vi "NEW TESTS 4 channel fixed pixel clock resonance scanner acquisition (Host).vi"() -> ()   [LabVIEW 2012]
uses:
  <vilib>/rvi/interface/nirviOpenFPGA/nirviOpenFPGA.xnode
  <vilib>/rvi/interface/nirviMethod/nirviMethod.xnode
  <vilib>/rvi/interface/nirviReadWriteControl/nirviReadWriteControl.xnode
  <vilib>/rvi/errors/niLvFpgaMergeErrorWithErrorCode.vi
  <vilib>/rvi/interface/nirviCloseFPGA/nirviCloseFPGA.xnode
  <vilib>/DAQmx/create/channels.llb/DAQmx Create Channel (AO-Voltage-Basic).vi
  <vilib>/DAQmx/configure/timing.llb/DAQmx Timing (Sample Clock).vi
  <vilib>/DAQmx/write.llb/DAQmx Write (Analog 1D DBL 1Chan NSamp).vi
  <vilib>/DAQmx/configure/trigger.llb/DAQmx Start Trigger (Digital Edge).vi
  D/Dropbox/Scientifica SoftScan project/fpga testing/4 ch resonance scanner acquisition (FPGA) fixed pix clock.vi
  Scientifica SoftScan project/fpga testing/FPGA Bitfiles/4chresonancescan_PXIe-7962R_newLindsaymod4ch_VaUfink3TSc.lvbitx
  <vilib>/userdefined/High Color/nirio_resource_hc.ctl
panel:
  in  "Numeric":i32=200
  out "Waveform Graph 2":i32[](graph)
  out "Array 4":i32[](array[numeric])
  out "sum 2":i16
  out "Array 3":u32[](array[numeric])
  out "max index(es)":i32
  out "Waveform Graph":u32[](graph)
  out "min value":u32
  out "max value":u32
  out "avg value":dbl
  out "sum":u32
  out "Array 2":u32[](array[numeric])
  out "Array":u32[](array[numeric])
  out "Waveform Chart":u32[](graph)
  out "Timed Out":bool
  out "Numeric 2":i32
  in  "data":dbl=1.0
  in  "y-voltage":dbl=4.0
  out "error out":errorcluster
  in  "stop":bool
  in  "Requested Depth":u32=100000000
  in  "lines (2pi) per frame":i32=100
  out "Actual Depth 3":u32
  out "Actual Depth":u32
  in  "Start Delay (Ticks)":i16
  in  "RIO Device":T1="RIO0"
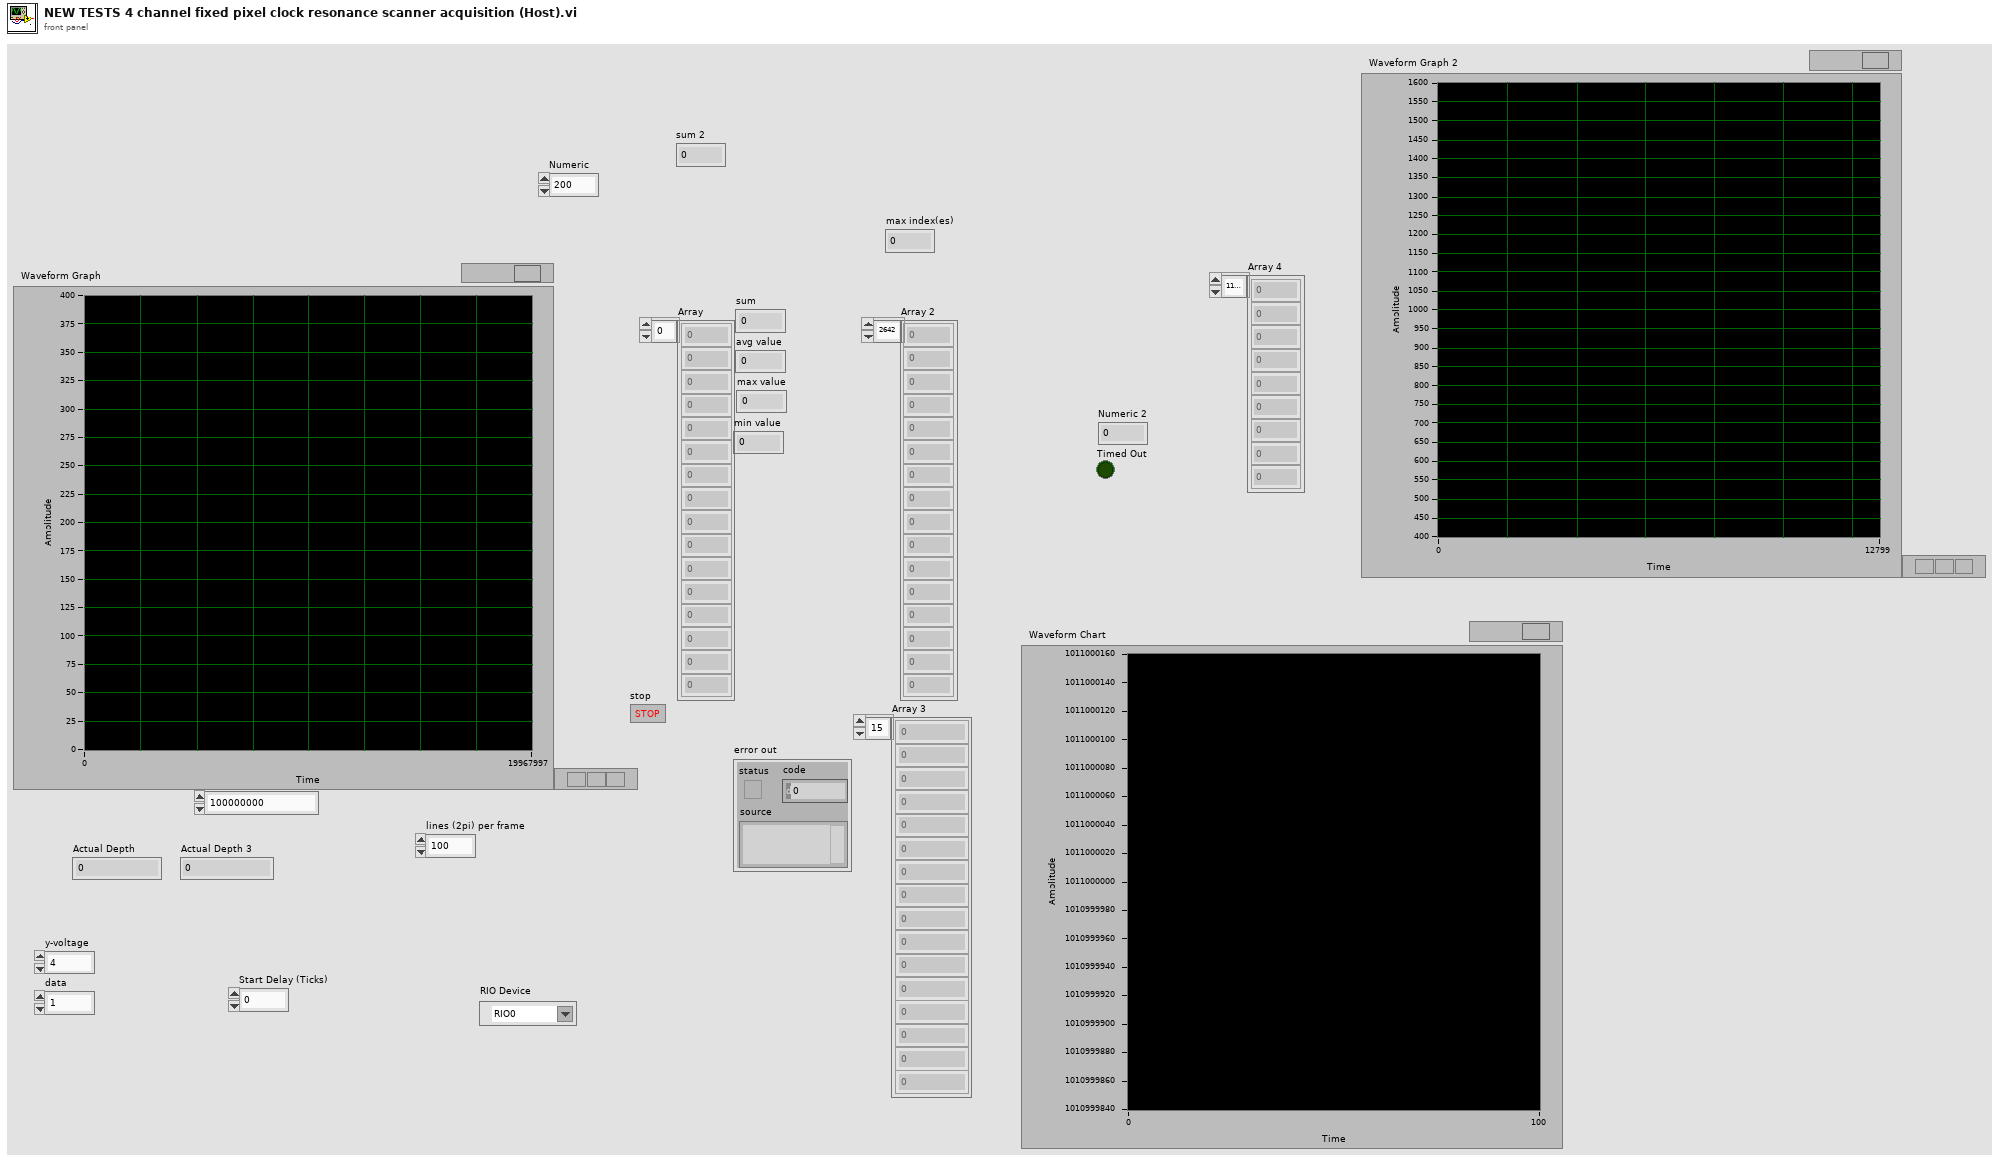
[diagram p1: front panel]
types:
  T1 = typedef "nirio_resource_hc.ctl" = tag
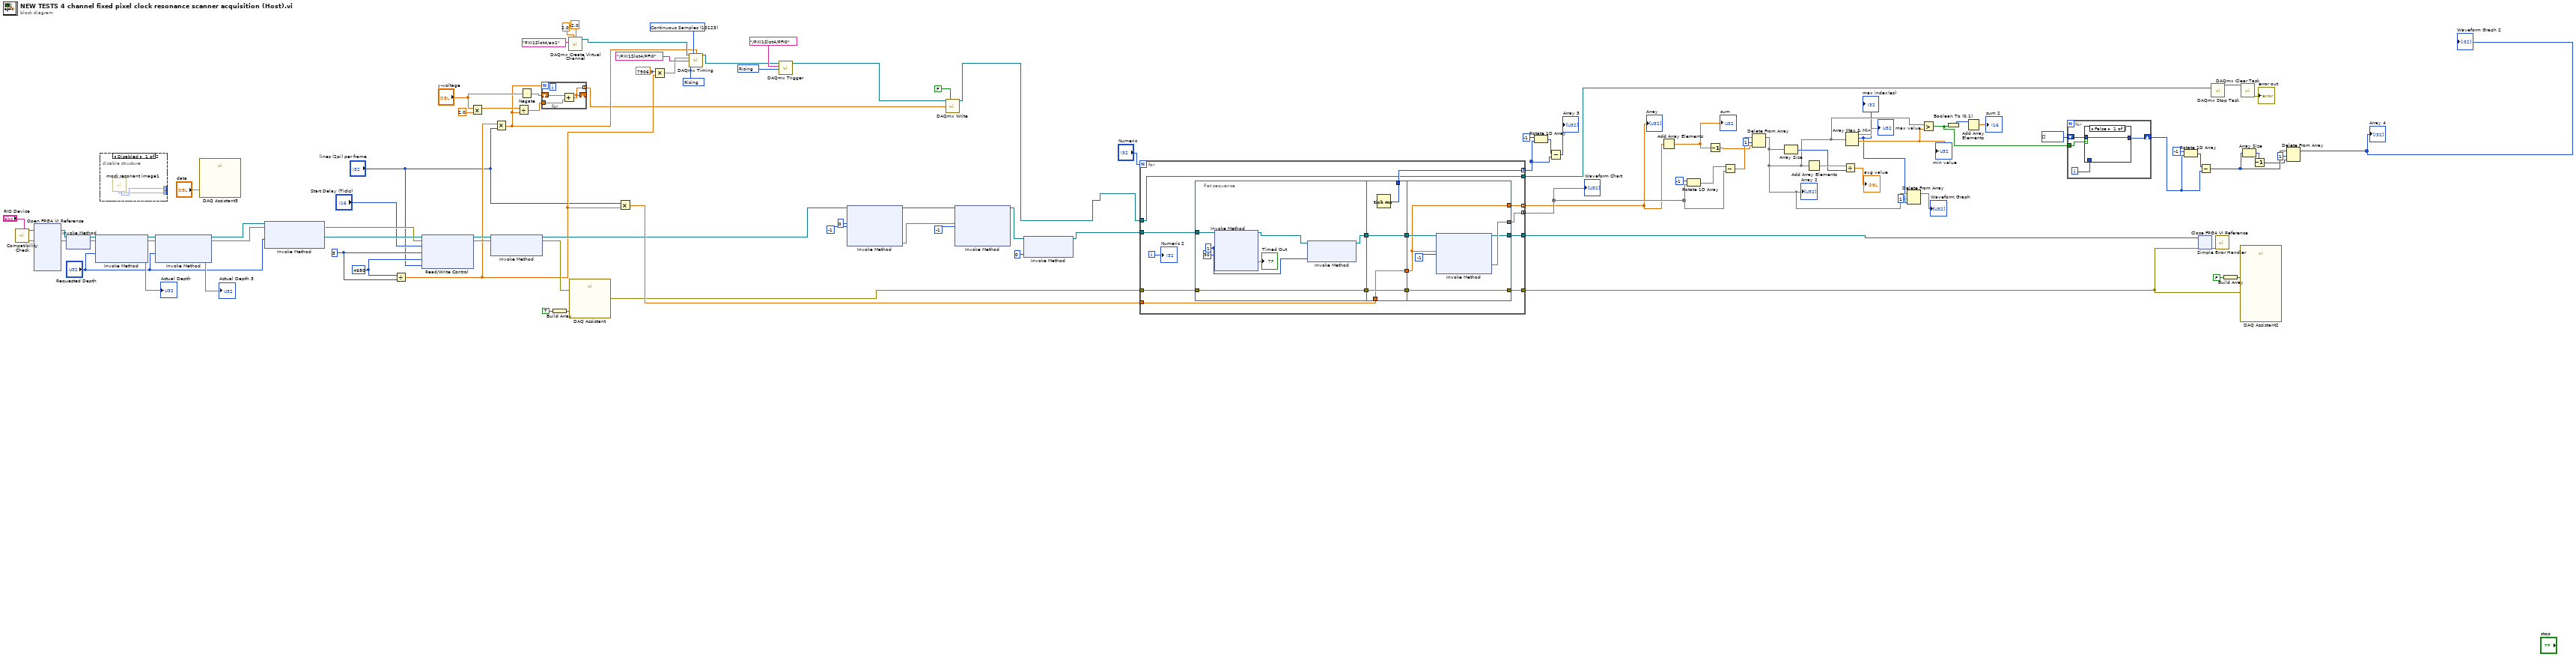
[diagram p0: block diagram]
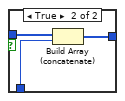
[diagram p2: hidden frame]
diagram:
  w10 = 10280 items=["Rising"=10280, "Falling"=10171] ("active edge")
  w75 = 10123 items=["Finite Samples"=10178, "Continuous Samples"=10123, "Hardware Timed Single Point"=12522] ("sample mode")
  w85 = 3 ("dwell time in ticks")
  w8 = i16 4680 ("samples per period")
  w89 = 10280 items=["Rising"=10280, "Falling"=10171] ("edge")
  n1 = call "Compatibility Check.vi"() -> ("error out"=w101:errorcluster)  [unwired: 2 in, 9 out]
  n2 = xnode "Open FPGA VI Reference"("error in"=w101, "resource name"="RIO Device") -> ("FPGA VI Reference Out"=w98:refnum<k20>, "error out"=w99:errorcluster)
  n3 = xnode "Invoke Method"("FPGA VI Reference In"=w98, "error in"=w99) -> ("FPGA VI Reference Out"=w97:refnum<k20>, "error out"=w88:errorcluster)
  n4 = xnode "Invoke Method"("FPGA VI Reference In"=w97, "error in"=w88, "Requested Depth"="Requested Depth") -> ("FPGA VI Reference Out"=w93:refnum<k20>, "error out"=w87:errorcluster, "Actual Depth"=→"Actual Depth")
  n5 = disable-structure shown="Disabled" {
    disable-tunnel: [w103 _] -> _
    disable-tunnel: [w102 _] -> _
    frame Disabled {
      n6 = call "mock resonant image1.vi"() -> ("samples per period (fix pix clock)"=w103:i32, "fixed dwell time"=w102:i32)  [unwired: 7 in, 3 out]
    }
    frame Enabled {
    }
  }
  n7 = xnode "Invoke Method"("FPGA VI Reference In"=w93, "error in"=w87, "Requested Depth"="Requested Depth") -> ("FPGA VI Reference Out"=w72:refnum<k20>, "error out"=w71:errorcluster, "Actual Depth"=→"Actual Depth 3")
  n8 = call "DAQ Assistant3"("data"="data") -> ()  [unwired: 17 in, 2 out]
  n9 = xnode "Invoke Method"("FPGA VI Reference In"=w72, "error in"=w71, "Requested Depth"="Requested Depth") -> ("FPGA VI Reference Out"=w70:refnum<k20>, "error out"=w69:errorcluster)  [unwired: 1 out]
  n10 = Divide(x=w8, y=w85) -> (x/y=w5:dbl)
  n11 = xnode "Read/Write Control"("FPGA VI Reference In"=w70, "error in"=w69, "Start Delay (Ticks)"="Start Delay (Ticks)", "dwell time in ticks"=w85, "samples per period"=w8, "lines at once"="lines (2pi) per frame") -> ("FPGA VI Reference Out"=w96:refnum<k20>, "error out"=w86:errorcluster)
  n12 = Multiply(x="y-voltage", y=2.0) -> (x*y=w12:dbl)
  n13 = xnode "Invoke Method"("FPGA VI Reference In"=w96, "error in"=w86) -> ("FPGA VI Reference Out"=w65:refnum<k20>, "error out"=w84:errorcluster)  [unwired: 1 in]
  n14 = Multiply(x=w5, y="lines (2pi) per frame") -> (x*y=w13:dbl)
  n15 = Divide(x=w12, y=w13) -> (x/y=w81:dbl)
  n16 = Negate(x="y-voltage") -> (-x=w80:dbl)
  n17 = for {
    N: w13 -> [_]
    tunnel: w81 -> [w105]
    shift-right: [w104] -> _
    shift-left: w80 -> [w106]
    tunnel: [w104] -> w2 mode=indexing
    n18 = Add(x=w106, y=w105) -> (x+y=w104:dbl)
  }
  n19 = Build Array(TRUE) -> (w91:bool[])
  n20 = call-poly <vilib>:"DAQmx Create Virtual Channel.vi"("maximum value"=2.0, "minimum value"=-2.0, "physical channels"=tag "PXI1Slot4/ao1") -> ("task out"=w83:refnum<k21>)  [unwired: 11 in, 1 out]
  n21 = call "DAQ Assistant"("data"=w91, "error in"=w84) -> ("error out"=w66:errorcluster)  [unwired: 16 in, 1 out]
  n22 = Multiply(x="lines (2pi) per frame", y=w5) -> (x*y=w67:dbl)
  n23 = Multiply(x=7906.0 ("rate"), y=w5) -> (x*y=w7:dbl)
  n24 = call-poly <vilib>:"DAQmx Timing.vi"("task/channels in"=w83, "sample mode"=w75, "samples per channel"=w13, "rate"=w7, "source"=tag "/PXI1Slot4/PFI0", "active edge"=w10) -> ("task out"=w9:refnum<k21>)  [unwired: 8 in, 1 out]
  n25 = call-poly <vilib>:"DAQmx Trigger.vi"("task/channels in"=w9, "source"=tag "/PXI1Slot4/PFI0", "edge"=w89) -> ("task out"=w4:refnum<k21>)  [unwired: 11 in, 1 out]
  n26 = xnode "Invoke Method"("FPGA VI Reference In"=w65, "Number of Elements"=u32 0, "Timeout (ms)"=-1) -> ("FPGA VI Reference Out"=w38:refnum<k20>, "Elements Remaining"=w37)  [unwired: 1 in, 2 out]
  n27 = call-poly <vilib>:"DAQmx Write.vi"("task/channels in"=w4, "auto start"=FALSE, "data"=w2) -> ("task out"=w3:refnum<k21>)  [unwired: 10 in, 2 out]
  n28 = xnode "Invoke Method"("FPGA VI Reference In"=w38, "Number of Elements"=w37, "Timeout (ms)"=-1) -> ("FPGA VI Reference Out"=w36:refnum<k20>)  [unwired: 1 in, 3 out]
  n29 = xnode "Invoke Method"("FPGA VI Reference In"=w36, "IRQ Number(s)"=0) -> ("FPGA VI Reference Out"=w54:refnum<k20>)  [unwired: 1 in, 1 out]
  n30 = for {
    N: "Numeric" -> [_]
    tunnel: [w112] -> w61
    tunnel: [w111] -> w60
    tunnel: [w108] -> w58
    tunnel: w66 -> [w121]
    tunnel: w3 -> [w108]
    tunnel: w67 -> [w107]
    tunnel: [w114] -> w50 mode=indexing
    tunnel: [w113] -> w51 mode=concatenating
    tunnel: w54 -> [w110]
    tunnel: [w109] -> w25 mode=indexing
    i -> [w120]
    n31 = flat-sequence {
      tunnel: w121 -> [w128]
      tunnel: [w128] -> w119
      tunnel: [w123] -> w118
      tunnel: w110 -> [w126]
      tunnel: w119 -> [w132]
      tunnel: [w132] -> w117
      tunnel: w118 -> [w130]
      tunnel: [w129] -> w116
      tunnel: [w130] -> w115
      tunnel: [w131] -> w109
      tunnel: w107 -> [w129]
      tunnel: w117 -> [w133]
      tunnel: w116 -> [w136]
      tunnel: w115 -> [w137]
      tunnel: [w136] -> w114
      tunnel: [w135] -> w113
      tunnel: [w134] -> w112
      tunnel: [w133] -> w111
      frame #0 {
        w125 = 1 ("IRQ Number(s)")
        n32 = xnode "Invoke Method"("FPGA VI Reference In"=w126, "IRQ Number(s)"=w125, "Timeout (ms)"=30) -> ("FPGA VI Reference Out"=w124:refnum<k20>, "Timed Out"=→"Timed Out")  [unwired: 1 in, 2 out]
        n33 = xnode "Invoke Method"("FPGA VI Reference In"=w124, "IRQ Number(s)"=w125) -> ("FPGA VI Reference Out"=w123:refnum<k20>)  [unwired: 1 in, 1 out]
      }
      frame #1 {
        n34 = Tick Count (ms)() -> (millisecond timer value=w131:u32)
      }
      frame #2 {
        n35 = xnode "Invoke Method"("FPGA VI Reference In"=w137, "Number of Elements"=w136, "Timeout (ms)"=-1) -> ("FPGA VI Reference Out"=w134:refnum<k20>, "Data"=w135:void[])  [unwired: 1 in, 2 out]
      }
    }
    "Numeric 2" <- w120
  }
  "Waveform Chart" <- w51
  "Array" <- w50
  n36 = Rotate 1D Array(1:w25, 2:-1 ("n")) -> (0:w26:u32[])
  n37 = Subtract(x=w26, y=w25) -> (x-y=→"Array 3":u32[])
  n38 = Add Array Elements(numeric array=w50) -> (sum=w43:dbl)
  "sum" <- w43
  n39 = Rotate 1D Array(1:w51, 2:-1 ("n")) -> (0:w52:void[])
  n40 = Decrement(x=w43) -> (x-1=w42:dbl)
  n41 = Subtract(x=w52, y=w51) -> (x-y=w48:dbl)
  n42 = Delete From Array(array=w48, length=1, index=w42) -> (array with subset deleted=w32)  [unwired: 1 out]
  "Array 2" <- w32
  n43 = Array Size(array=w32) -> (size(s)=w46:i32)
  n44 = Add Array Elements(numeric array=w32) -> (sum=w47:dbl)
  n45 = Divide(x=w47, y=w46) -> (x/y=→"avg value":dbl)
  n46 = Array Max & Min(array=w32) -> (max value=→"max value":dbl, max index (indices)=w31:i32, min value=w35:dbl)  [unwired: 1 out]
  "min value" <- w35
  "max index(es)" <- w31
  n47 = Delete From Array(array=w32, length=1, index=w31) -> (array with subset deleted=→"Waveform Graph")  [unwired: 1 out]
  n48 = Greater?(x=w32, y=w35) -> (0:w24:bool)
  n49 = Boolean To (0,1)(Boolean=w24) -> (0, 1=w34:i16)
  n50 = Add Array Elements(numeric array=w34) -> (sum=→"sum 2":dbl)
  n51 = for {
    tunnel: w24 -> [w139]
    shift-right: [w141] -> w20
    shift-left: i32[] [] -> [w140]
    i -> [w142]
    n52 = case shown="False" w139 {
      tunnel: w142 -> [_ w146]
      tunnel: [w143 w145] -> w141
      tunnel: w140 -> [w143 w144]
      frame False {
      }
      frame True {
        n53 = Build Array (concatenate)(w144, w146) -> (w145:i32[])
      }
    }
  }
  n54 = Rotate 1D Array(1:w20, 2:-1 ("n")) -> (0:w22:i32[])
  n55 = xnode "Close FPGA VI Reference"("FPGA VI Reference In"=w61, "error in"=w60) -> ("error out"=w62:errorcluster)
  n56 = Subtract(x=w22, y=w20) -> (x-y=w19:i32[])
  n57 = call <vilib>:"DAQmx Stop Task.vi"("task/channels in"=w58) -> ("task out"=w57:refnum<k21>)  [unwired: 13 in, 1 out]
  n58 = call <vilib>:"Simple Error Handler.vi"("error in (no error)"=w62) -> ()  [unwired: 1 in, 8 out]
  n59 = Build Array(FALSE) -> (w64:bool[])
  n60 = call "DAQ Assistant2"("data"=w64, "error in"=w60) -> ()  [unwired: 16 in, 2 out]
  n61 = call <vilib>:"DAQmx Clear Task.vi"("task in"=w57) -> ("error out"=→"error out":errorcluster)  [unwired: 14 in]
  n62 = Array Size(array=w19) -> (size(s)=w18:i32)
  n63 = Decrement(x=w18) -> (x-1=w15:i32)
  n64 = Delete From Array(array=w19, length=1, index=w15) -> (array with subset deleted=→"Array 4" →"Waveform Graph 2":i32[])  [unwired: 1 out]
